vi "界面UI.vi"() -> ()   [LabVIEW 2016, in "超标留样集成.lvlib" / "德润DR803M超标留样.lvlib"]
uses:
  <vilib>/Utility/miscctls.llb/LVPointTypeDef.ctl
  <vilib>/Utility/config.llb/NI_LVConfig.lvlib
panel:
  out "String":string
  in  "超标测试":bool
  out "超标留样信号":bool
  out "留样结果":bool
  in  "协议选择":enum16{"原始协议", "MODBUS协议"}(ring)
  in  "设置":bool
  in  "工作进程":u16(ring) items=["停止中"=0, "启动延时"=1, "外置泵延时"=2, "管路润洗"=3, "管存"=4, "留样"=5, "出水管路排空"=6, "采水管路排空"=7, "待机"=13]
  out "采样器进程":i32(listbox)
  out "采样瓶数":u16
  out "留样模式":T1(ring)
  out "门状态":enum16{"门关", "门开"}(ring)
  out "仪器时间":timestamp format="%<%Y/%m/%d %H:%M:%S>T"
  out "当前瓶号":u16
  out "采样器状态":enum16{"停止", "运行", "系统初始化"}(ring)
  out "留样瓶满报警":bool
  out "超标留样等待时间/s":dbl
  in  "流程停止":bool
  in  "流程启动":bool
  out "流程中":bool
  out "VISA resource name":refnum<visa-resource-name>="COM10" caption="VISA资源名称"
  in  "采样启动":bool
  in  "切换运行":bool
  in  "时间校准":bool
  out "source":string
  out "通讯":bool
  # "只在待机时启动有效"
  # "德润超标留样803M"
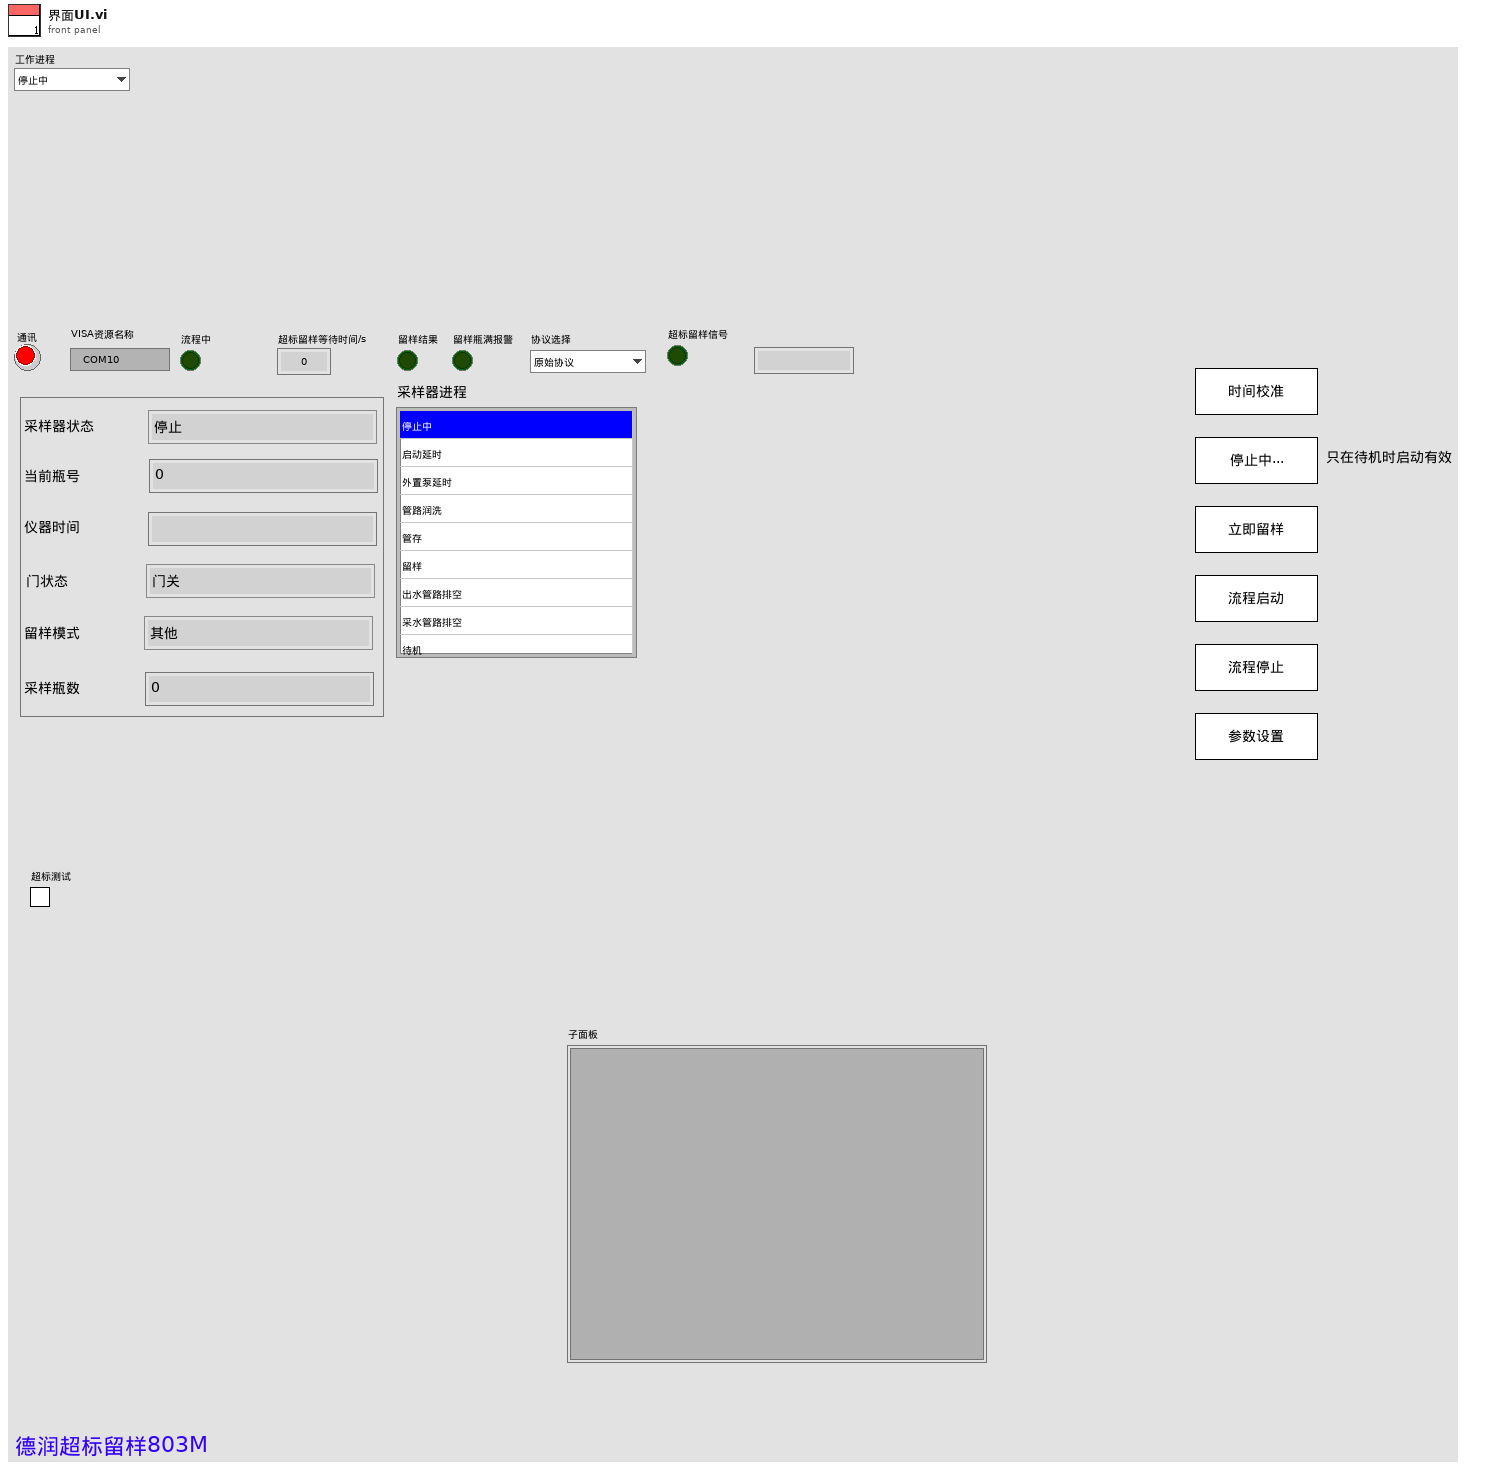
[diagram p1: front panel]
types:
  T1 = enum16{"其他", "定时留样", "时间等比例", "同步留样", "外控留样", "超标留样"}
  T2 = typedef "超标留样集成.lvlib/德润DR803M超标留样.lvlib/typedef.ctl" = cluster{"枚举":enum16{"open", "read", "write", "close", "write_register"}, "写入内容":string, "data_in":cluster{"write_coil_in":cluster{"address":u16, "value":bool}, "write_register_in":cluster{"address":u16, "values":u16[]}, "read_register_in":cluster{"starting address":u16, "quantity":u16}}}
  T3 = typedef "LVPointTypeDef.ctl" = cluster{"Horizontal":i16, "Vertical":i16}
  T4 = enum16{"打开串口", "写入", "读取", "关闭串口", "写入寄存器", "读取线圈"}
  T5 = cluster{"write_coil_in":cluster{"address":u16, "value":bool}, "write_register_in":cluster{"address":u16, "values":u16[]}, "read_register_in":cluster{"starting address":i32, "quantity":u16}}
  T6 = cluster{"write_coil_in":cluster{"address":u16, "value":bool}, "write_register_in":cluster{"address":u16, "values":u16[]}, "read_register_in":cluster{"starting address":u16, "quantity":u16}}[]
  T7 = cluster{"采样器状态":enum16{"停止", "运行", "系统初始化-2", "系统初始化-3", "初始化失败"}, "仪器时间":timestamp, "留样结果":bool, "工作模式":u16, "当前瓶号":u16, "平行样数":u16, "采样瓶数":u16, "设定每瓶采样次数":u16, "每瓶采样量":u16, "当前进程":u16, "当前瓶已采次数":u16, "留样中":bool}
  T8 = cluster{"仪器时间":timestamp, "工作状态":u16, "工作进程":u16, "采样模式":u16, "采样瓶数":dbl, "当前瓶号":dbl, "设定平行样数":dbl, "已采平行样":dbl, "设定每瓶采样次数":dbl, "已采次数":dbl, "当前瓶采样量":dbl, "瞬时流量":dbl, "累积流量":dbl, "混匀桶已采次数":dbl, "COD":dbl, "NH3N":dbl, "门状态":u16, "采样泵使能":dbl, "采样泵方向":dbl, "导流电机使能":dbl, "导流电机方向":dbl, "阀A":dbl, "阀B":dbl, "阀C":dbl, "外置泵":dbl, "预留":dbl}
  T9 = enum16{"停止", "运行", "系统初始化-2", "系统初始化-3", "初始化失败"}
  T10 = enum16{"open", "read", "write", "close", "write_register"}
  T11 = cluster{"write_coil_in":cluster{"address":u16, "value":bool}, "write_register_in":cluster{"address":u16, "values":u16[]}, "read_register_in":cluster{"starting address":u16, "quantity":u16}}
  T12 = typedef "LVDateTimeRec.ctl" = cluster{"秒数的小数部分":dbl, "秒":i32, "分":i32, "时":i32, "日":i32, "月":i32, "年":i32, "天数（周）":i32, "天数（年）":i32, "DST":i32}
  T13 = typedef "NI_LVConfig.lvlib/Config Data RefNum.ctl" = refnum<k1>
  T14 = enum32{"Bad", "Idle", "Run top level", "Running"}
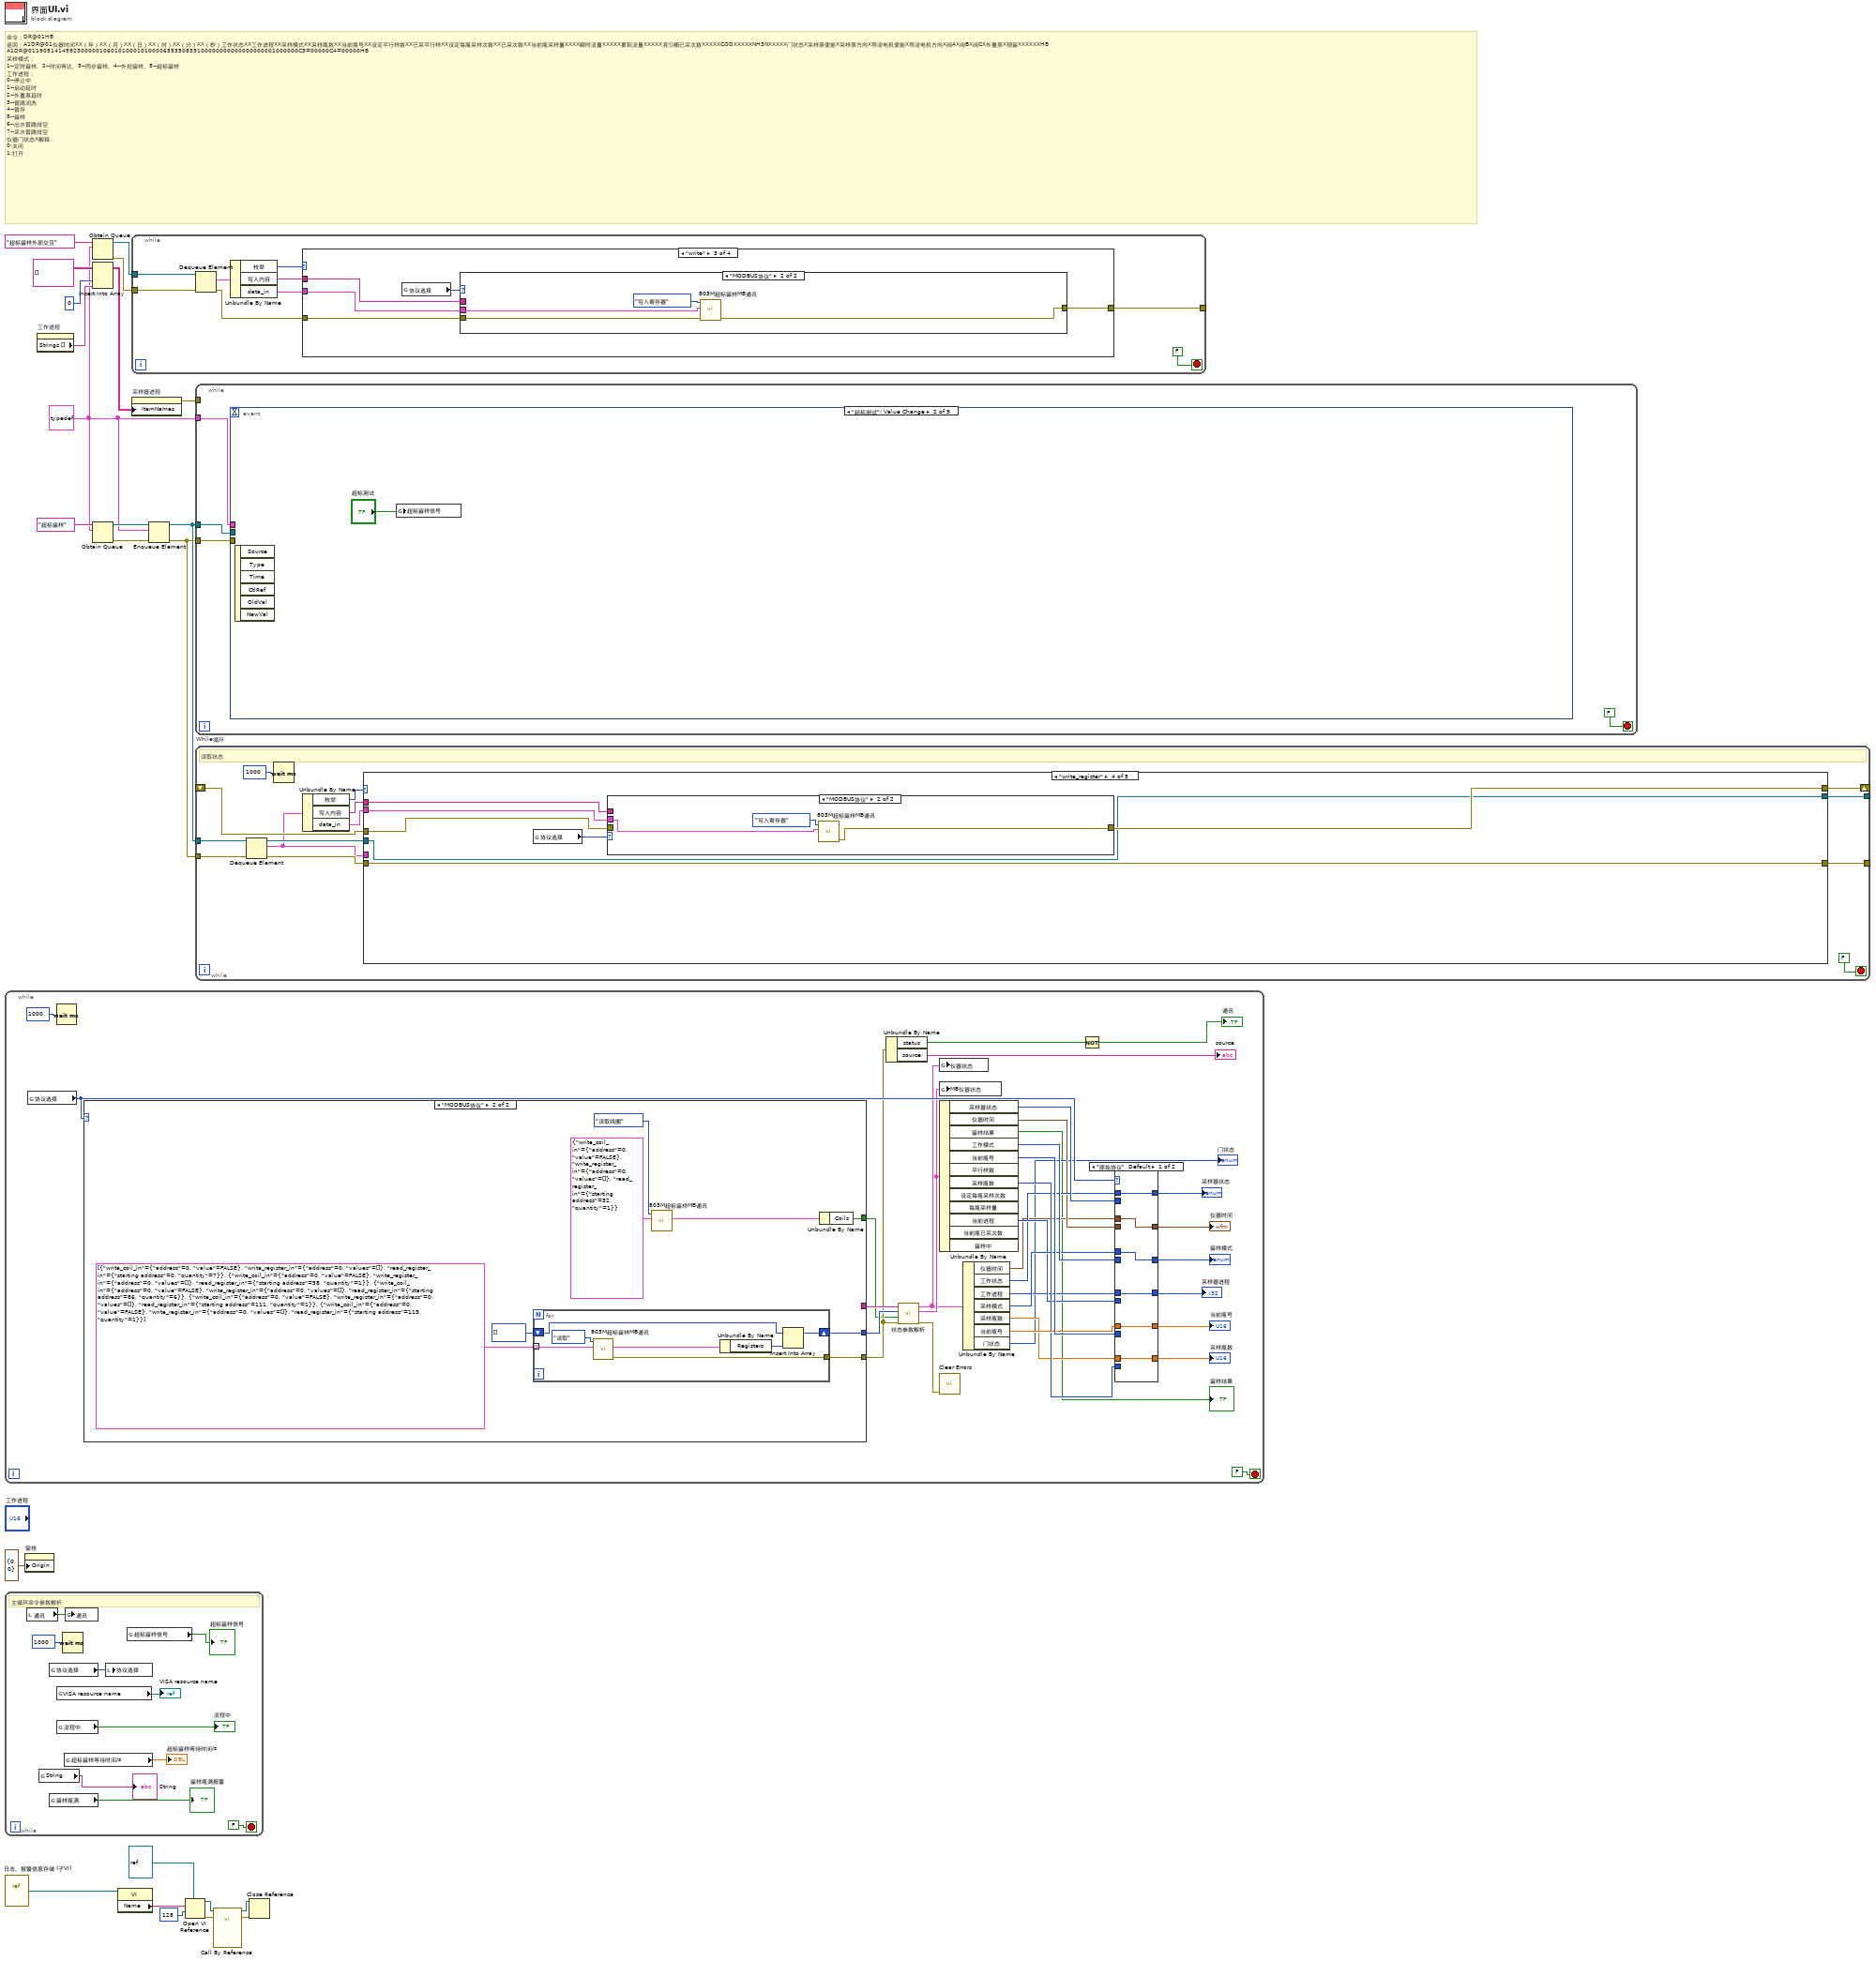
[diagram p0: block diagram]
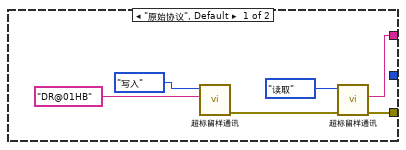
[diagram p3: hidden frame]
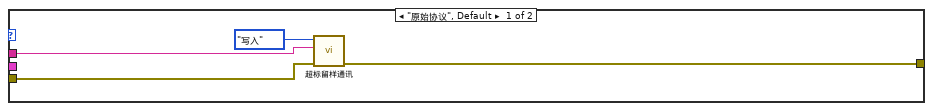
[diagram p6: hidden frame]
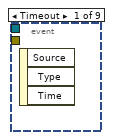
[diagram p8: hidden frame]
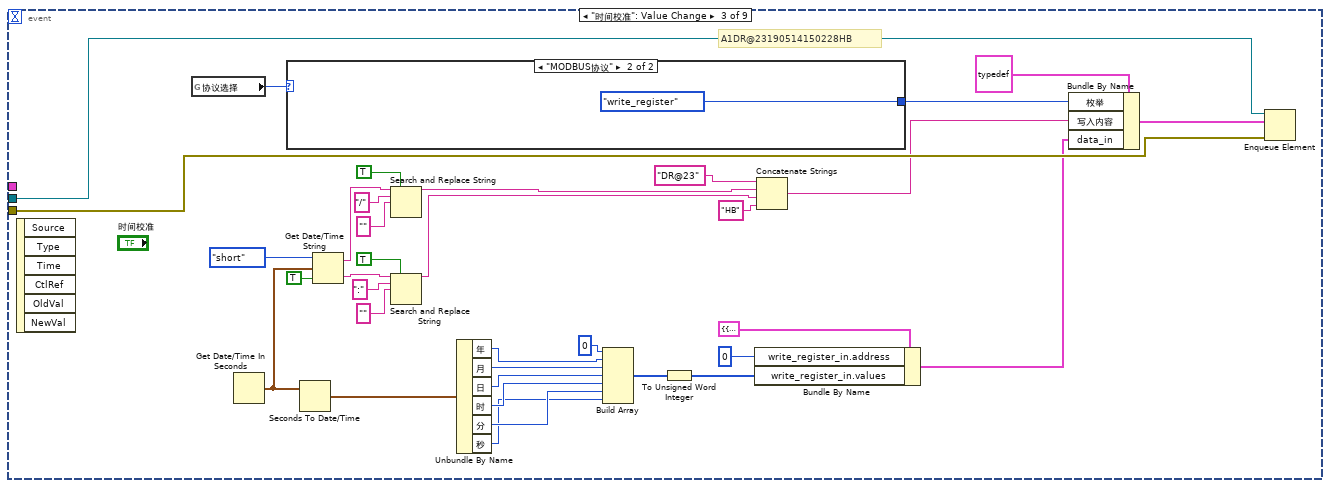
[diagram p9: hidden frame]
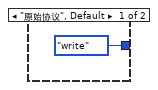
[diagram p10: hidden frame]
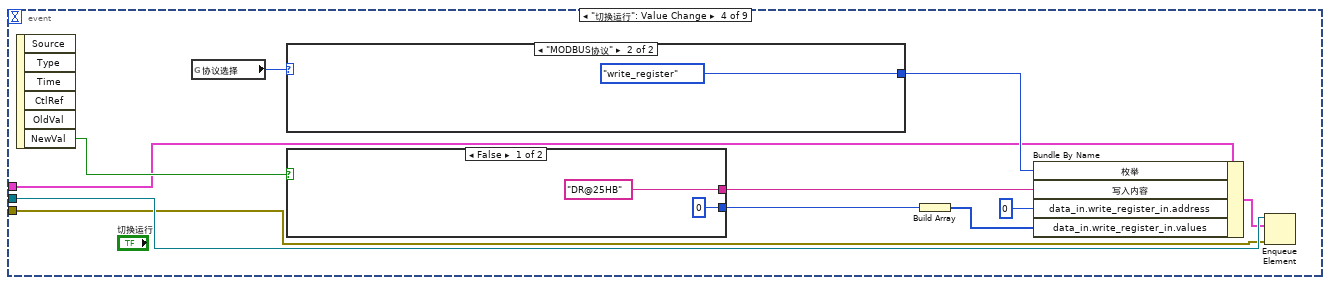
[diagram p11: hidden frame]
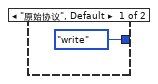
[diagram p12: hidden frame]
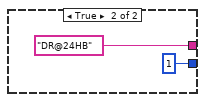
[diagram p13: hidden frame]
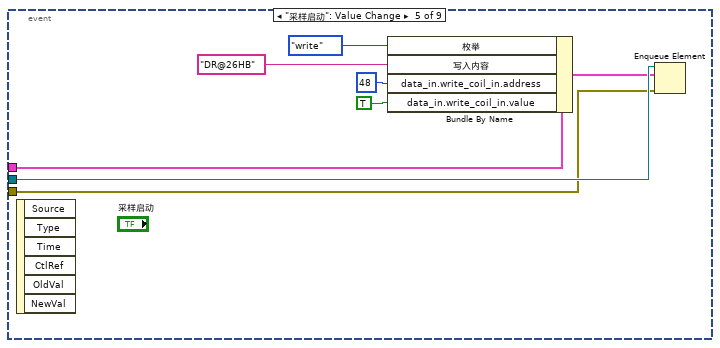
[diagram p14: hidden frame]
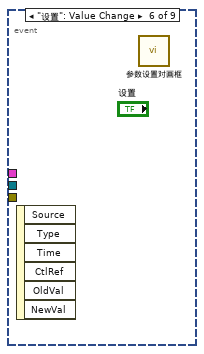
[diagram p15: hidden frame]
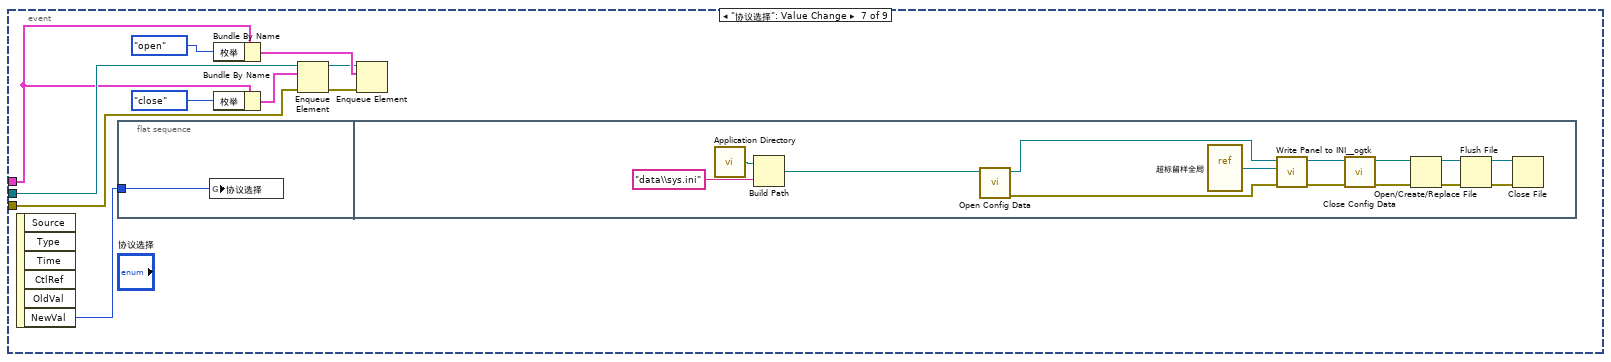
[diagram p16: hidden frame]
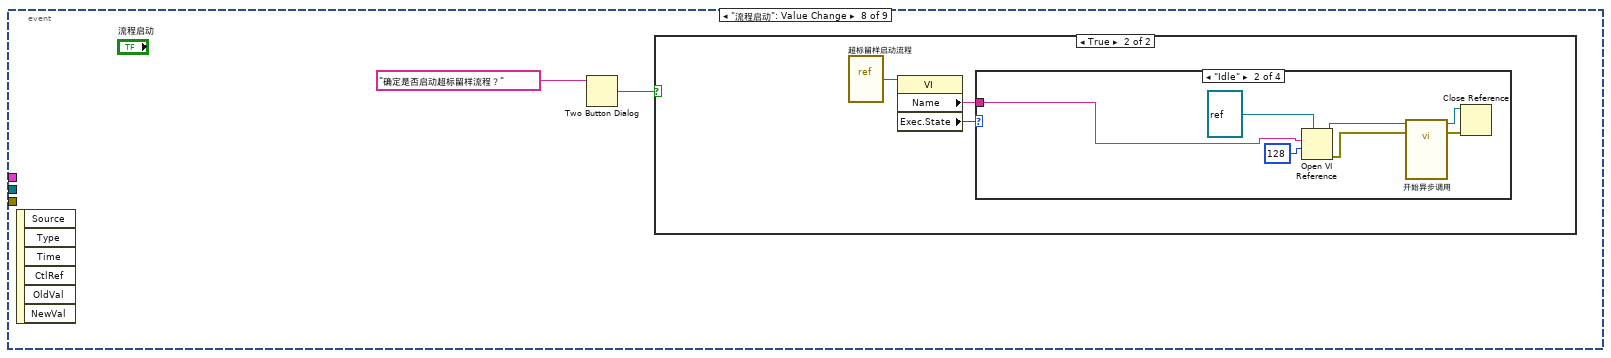
[diagram p17: hidden frame]
diagram:
  w1 = T2 {"枚举"=enum."open", "写入内容"="超标留样", "data_in"={"write_coil_in"={"address"=0, "value"=FALSE}, "write_register_in"={"address"=0, "values"=[]}, "read_register_in"={"starting address"=0, "quantity"=0}}}
  # "命令：DR@01HB\n返回：A1DR@01仪器时间XX（年）XX（月）XX（日）XX（时）XX（分）XX（秒）工作状态XX工作进程XX采样模式XX采样瓶数XX当前瓶号XX设定平行样数XX已采平行样XX设定每瓶采样次数XX已采次数XX当前瓶采样量XXXX瞬时流量XXXXX累积流量XXXXX混匀桶已采次数XXXXXCODXXXXXNH3NXXXXX门状态X采样泵使能X采样泵方向X导流电机使能X导流电机方向X阀AX阀BX阀CX外置泵X预留XXXXXXHB\nA1DR@011905141459230000010601010001010000655350839100000000000000000001000000C3=00000C4=00000HB\n采样模式：\n1--定时留样、2--时间等比、3--同步留样、4--外控留样、5--超标留样\n工作进程：\n0--停止中\n1--启动延时\n2--外置泵延时\n3--管路润洗\n4--管存\n5--留样\n6--出水管路排空\n7--采水管路排空\n仪器门状态X解释：\n0:关闭\n1:打开"
  n1 = while {
    stop <- FALSE stop-if-true
    n2 = global read "超标留样全局.vi" "协议选择"() -> (w39:enum16{"原始协议", "MODBUS协议"})
    n3 = Wait (ms)(milliseconds to wait=u32 1000 ("等待时间（毫秒）")) -> ()  [unwired: 1 out]
    n4 = case shown="\"MODBUS协议\"" w39 {
      tunnel: [w73 w79] -> w27
      tunnel: [w72 _] -> w28
      tunnel: [_ w80] -> w34
      tunnel: [_ w75] -> w24
      frame "原始协议", Default {
        n5 = call "超标留样通讯.vi"("写入缓冲区"="DR@01HB", "功能输入"=enum16{"打开串口", "写入", "读取", "关闭串口"}."写入") -> ("error out"=w74:errorcluster)  [unwired: 7 in, 2 out]
        n6 = call "超标留样通讯.vi"("error in (no error)"=w74, "功能输入"=enum16{"打开串口", "写入", "读取", "关闭串口"}."读取") -> ("error out"=w73:errorcluster, "读取缓冲区"=w72:string)  [unwired: 7 in, 1 out]
      }
      frame "MODBUS协议" {
        n7 = for {
          shift-right: [w86] -> w80
          shift-left: u16[] [] -> [w85]
          tunnel: T6 [{"write_coil_in"={"address"=0, "value"=FALSE}, "write_register_in"={"address"=0, "values"=[]}, "read_register_in"={"starting address"=0, "quantity"=7}}, {"write_coil_in"={"address"=0, "value"=FALSE}, "write_register_in"={"address"=0, "values"=[]}, "read_register_in"={"starting address"=58, "quantity"=1}}, {"write_coil_in"={"address"=0, "value"=FALSE}, "write_register_in"={"address"=0, "values"=[]}, "read_register_in"={"starting address"=86, "quantity"=6}}, {"write_coil_in"={"address"=0, "value"=FALSE}, "write_register_in"={"address"=0, "values"=[]}, "read_register_in"={"starting address"=111, "quantity"=1}}, {"write_coil_in"={"address"=0, "value"=FALSE}, "write_register_in"={"address"=0, "values"=[]}, "read_register_in"={"starting address"=115, "quantity"=1}}] -> [w84] mode=indexing
          tunnel: [w83] -> w79
          n8 = call "803M超标留样MB通讯.vi"("data_in"=w84, "功能输入"=T4."读取") -> ("error out"=w83:errorcluster, "data_out"=w88:cluster{"Registers":u16[], "Coils":bool[]})  [unwired: 8 in]
          n9 = Unbundle By Name(w88) -> ("Registers"=w87:u16[])
          n10 = Insert Into Array(array=w85, new element=w87) -> (w86:u16[])  [unwired: 1 in]
        }
        n11 = call "803M超标留样MB通讯.vi"("data_in"=T5 {"write_coil_in"={"address"=0, "value"=FALSE}, "write_register_in"={"address"=0, "values"=[]}, "read_register_in"={"starting address"=32, "quantity"=1}}, "功能输入"=T4."读取线圈") -> ("data_out"=w76:cluster{"Registers":u16[], "Coils":bool[]})  [unwired: 8 in, 1 out]
        n12 = Unbundle By Name(w76) -> ("Coils"=w75:bool[])
      }
    }
    n13 = Unbundle By Name(w27) -> ("status"=w29:bool, "source"=→"source":string)
    n14 = call "状态参数解析.vi"("error in (no error)"=w27, "Coils"=w24, "数组"=w34, "字符串"=w28) -> ("error out"=w33:errorcluster, "簇 2"=w35:T7, "簇"=w32:T8)  [unwired: 5 in]
    n15 = global write "超标留样全局.vi" "仪器状态"(w32) -> ()
    n16 = global write "超标留样全局.vi" "MB仪器状态"(w35) -> ()
    n17 = Unbundle By Name(w35) -> ("采样器状态"=w43:T9, "仪器时间"=w40:timestamp, "留样结果"=→"留样结果":bool, "工作模式"=w49:u16, "当前瓶号"=w55:u16, "采样瓶数"=w52:u16, "当前进程"=w46:u16)  [unwired: 5 out]
    n18 = call <vilib>:"Clear Errors.vi"("error in (no error)"=w33) -> ()  [unwired: 5 in, 2 out]
    n19 = Unbundle By Name(w32) -> ("仪器时间"=w37:timestamp, "工作状态"=w41:u16, "工作进程"=w44:u16, "采样模式"=w47:u16, "采样瓶数"=w50:dbl, "当前瓶号"=w53:dbl, "门状态"=→"门状态":u16)
    n20 = Not(x=w29) -> (.not. x?=→"通讯":bool)
    n21 = case shown="\"原始协议\", Default" w39 {
      tunnel: w37 -> [w62 _]
      tunnel: [w62 w68] -> w38
      tunnel: w40 -> [_ w68]
      tunnel: w41 -> [w61 _]
      tunnel: [w61 w67] -> w42
      tunnel: w43 -> [_ w67]
      tunnel: w44 -> [w60 _]
      tunnel: [w60 w66] -> w45
      tunnel: w46 -> [_ w66]
      tunnel: w47 -> [w59 _]
      tunnel: [w59 w65] -> w48
      tunnel: w49 -> [_ w65]
      tunnel: w50 -> [w58 _]
      tunnel: [w58 w64] -> w51
      tunnel: w52 -> [_ w64]
      tunnel: w53 -> [w57 _]
      tunnel: [w57 w63] -> w54
      tunnel: w55 -> [_ w63]
      frame "原始协议", Default {
      }
      frame "MODBUS协议" {
      }
    }
    "仪器时间" <- w38
    "采样器状态" <- w42
    "当前瓶号" <- w54
    "留样模式" <- w48
    "采样瓶数" <- w51
    "采样器进程" <- w45
  }
  n22 = while {
    stop <- FALSE stop-if-true
    # "主循环命令参数解析"
    n23 = local read "通讯"() -> (w97:bool)
    n24 = global read "超标留样全局.vi" "String"() -> (→"String":string)
    n25 = global read "超标留样全局.vi" "协议选择"() -> (w92:enum16{"原始协议", "MODBUS协议"})
    n26 = global read "超标留样全局.vi" "留样瓶满"() -> (→"留样瓶满报警":bool)
    n27 = global read "超标留样全局.vi" "VISA resource name"() -> (→"VISA resource name":refnum<visa-resource-name>)
    n28 = global read "超标留样全局.vi" "流程中"() -> (→"流程中":bool)
    n29 = Wait (ms)(milliseconds to wait=u32 1000 ("等待时间（毫秒）")) -> ()  [unwired: 1 out]
    n30 = global read "超标留样全局.vi" "超标留样等待时间/s"() -> (→"超标留样等待时间/s":dbl)
    n31 = global write "超标留样全局.vi" "通讯"(w97) -> ()
    n32 = local write "协议选择"(w92) -> ()
    n33 = global read "超标留样全局.vi" "超标留样信号"() -> (→"超标留样信号":bool)
  }
  n34 = vi-ref "日志、报警信息存储 (子VI).vi"() -> (w14:refnum<vi>)
  n35 = property on="窗格" class="Pane"("Origin"=T3 {"Horizontal"=0, "Vertical"=0} ("原点")) -> ()  [unwired: 2 in, 2 out]
  n36 = property on="工作进程" class="Ring (strict)"() -> ("Strings []"=w4:string[])  [unwired: 2 in, 2 out]
  n37 = Obtain Queue(name (unnamed)="超标留样外部交互" ("名称（未命名）"), element data type=w1) -> (queue out=w16:refnum<queue>, error out=w15:errorcluster)  [unwired: 3 in, 1 out]
  n38 = Insert Into Array(array=string[][] [] ("字符串[]"), index (col)=0 ("禁用的索引 (列)"), new element=w4) -> (w3:string[][])  [unwired: 1 in]
  n39 = Obtain Queue(name (unnamed)="超标留样" ("名称（未命名）"), element data type=w1) -> (queue out=w22:refnum<queue>, error out=w21:errorcluster)  [unwired: 3 in, 1 out]
  n40 = property class="VI"(reference=w14) -> ("Name"=w13:string)  [unwired: 1 in, 2 out]
  n41 = while {
    tunnel: w16 -> [w108]
    tunnel: w15 -> [w107]
    tunnel: [w101] -> _
    stop <- FALSE stop-if-true
    n42 = Dequeue Element(queue=w108, error in (no error)=w107) -> (element=w105:T2, error out=w102:errorcluster)  [unwired: 1 in, 2 out]
    n43 = Unbundle By Name(w105) -> ("枚举"=w104:T10, "写入内容"=w103:string, "data_in"=w100:T11)
    n44 = case shown="\"write\"" w104 {
      tunnel: w103 -> [_ _ w113 _]
      tunnel: w102 -> [_ _ w112 _]
      tunnel: [_ _ w111 _] -> w101
      tunnel: w100 -> [_ _ w109 _]
      frame "open", Default {
      }
      frame "read" {
      }
      frame "write" {
        n45 = global read "超标留样全局.vi" "协议选择"() -> (w110:enum16{"原始协议", "MODBUS协议"})
        n46 = case shown="\"MODBUS协议\"" w110 {
          tunnel: w113 -> [w117 _]
          tunnel: w112 -> [w115 w119]
          tunnel: [w114 w118] -> w111
          tunnel: w109 -> [_ w120]
          frame "原始协议", Default {
            n47 = call "超标留样通讯.vi"("error in (no error)"=w115, "写入缓冲区"=w117, "功能输入"=enum16{"打开串口", "写入", "读取", "关闭串口"}."写入") -> ("error out"=w114:errorcluster)  [unwired: 6 in, 2 out]
          }
          frame "MODBUS协议" {
            n48 = call "803M超标留样MB通讯.vi"("error in (no error)"=w119, "data_in"=w120, "功能输入"=enum16{"打开串口", "写入", "读取", "关闭串口", "写入寄存器"}."写入寄存器") -> ("error out"=w118:errorcluster)  [unwired: 7 in, 1 out]
          }
        }
      }
      frame "close" {
      }
    }
  }
  n49 = property on="采样器进程" class="MCListbox (strict)"("ItemNames"=w3) -> (error out=w2:errorcluster)  [unwired: 2 in, 1 out]
  n50 = Enqueue Element(queue=w22, element=w1, error in (no error)=w21) -> (queue out=w20:refnum<queue>, error out=w19:errorcluster)  [unwired: 1 in, 1 out]
  n51 = Open VI Reference(type specifier VI Refnum (for type only)=refnum<vi> refnum ("类型说明符VI引用句柄（仅用于类型）"), vi path=w13, options=128 ("选项")) -> (vi reference=w11:refnum<vi>, error out=w9:errorcluster)  [unwired: 3 in]
  n52 = while {
    tunnel: w20 -> [w124]
    tunnel: w19 -> [w123]
    tunnel: w2 -> [_]
    tunnel: w1 -> [w122]
    stop <- FALSE stop-if-true
    n53 = event shown="[1] \"超标测试\": Value Change" {
      selector: _ -> [_ _ _ _ _ _ _ _ _]
      dyn-events: _ -> [_ _ _ _ _ _ _ _ _]
      timeout: _ -> [_ _ _ _ _ _ _ _ _]
      tunnel: w124 -> [_ _ w161 w174 w188 _ w194 _ w228]
      tunnel: w123 -> [_ _ w160 w173 w187 _ w192 _ w227]
      tunnel: w122 -> [_ _ _ w168 w184 _ w193 _ w226]
      event Timeout {
        n54 = event-data() -> ()  [unwired: 1 in, 3 out]
      }
      event "超标测试": Value Change {
        n55 = event-data() -> ()  [unwired: 1 in, 6 out]
        n56 = global write "超标留样全局.vi" "超标留样信号"("超标测试") -> ()
      }
      event "时间校准": Value Change {
        # "A1DR@23190514150228HB"
        n57 = event-data() -> ()  [unwired: 1 in, 6 out]
        n58 = global read "超标留样全局.vi" "协议选择"() -> (w141:enum16{"原始协议", "MODBUS协议"})
        n59 = Get Date/Time In Seconds() -> (seconds since 1Jan1904=w138:timestamp)
        n60 = case shown="\"MODBUS协议\"" w141 {
          tunnel: [T10."write" ("枚举") T10."write_register" ("枚举")] -> w140
          frame "原始协议", Default {
          }
          frame "MODBUS协议" {
          }
        }
        n61 = Seconds To Date/Time(time stamp (now)=w138) -> (date time rec=w137:T12)  [unwired: 1 in]
        n62 = Get Date/Time String(date format (0)=enum16{"short", "long", "abbreviated"}."short" ("日期格式(0)"), seconds (now)=w138, want seconds? (F)=TRUE ("需要秒？(F)")) -> (date string=w156:string, time string=w149:string)
        n63 = Search and Replace String(replace all?=TRUE ("替换全部？(F)"), input string=w156, search string="/" ("搜索字符串"), replace string="" ("替换字符串(\"\")")) -> (result string=w148:string)  [unwired: 4 in, 3 out]
        n64 = Search and Replace String(replace all?=TRUE ("替换全部？(F)"), input string=w149, search string=":" ("搜索字符串"), replace string="" ("替换字符串(\"\")")) -> (result string=w147:string)  [unwired: 4 in, 3 out]
        n65 = Unbundle By Name(w137) -> ("年"=w136:i32, "月"=w135:i32, "日"=w134:i32, "时"=w133:i32, "分"=w132:i32, "秒"=w131:i32)
        n66 = Build Array(0 ("元素"), w136, w135, w134, w133, w132, w131) -> (w130:i32[])
        n67 = To Unsigned Word Integer(number=w130) -> (unsigned 16bit integer=w128:u16[])
        n68 = Bundle By Name(cluster=T11 {"write_coil_in"={"address"=0, "value"=FALSE}, "write_register_in"={"address"=0, "values"=[]}, "read_register_in"={"starting address"=0, "quantity"=0}} ("data_in"), "write_register_in.address"=u16 0, "write_register_in.values"=w128) -> (w139:T11)
        n69 = Concatenate Strings("DR@23" ("写入缓冲区"), w148, w147, "HB" ("写入缓冲区")) -> (w144:string)
        n70 = Bundle By Name(cluster=T2 {"枚举"=enum."open", "写入内容"="超标留样", "data_in"={"write_coil_in"={"address"=0, "value"=FALSE}, "write_register_in"={"address"=0, "values"=[]}, "read_register_in"={"starting address"=0, "quantity"=0}}}, "枚举"=w140, "写入内容"=w144, "data_in"=w139) -> (w145:T2)
        n71 = Enqueue Element(queue=w161, element=w145, error in (no error)=w160) -> ()  [unwired: 1 in, 3 out]
      }
      event "切换运行": Value Change {
        n72 = event-data() -> ("NewVal"=w172:bool)  [unwired: 1 in, 5 out]
        n73 = global read "超标留样全局.vi" "协议选择"() -> (w167:enum16{"原始协议", "MODBUS协议"})
        n74 = case shown="\"MODBUS协议\"" w167 {
          tunnel: [T10."write" ("枚举") T10."write_register" ("枚举")] -> w171
          frame "原始协议", Default {
          }
          frame "MODBUS协议" {
          }
        }
        n75 = case shown="False" w172 {
          tunnel: ["DR@25HB" ("写入缓冲区") "DR@24HB"] -> w170
          tunnel: [u16 0 ("value") u16 1 ("value")] -> w165
          frame False {
          }
          frame True {
          }
        }
        n76 = Build Array(w165) -> (w164:u16[])
        n77 = Bundle By Name(cluster=w168, "枚举"=w171, "写入内容"=w170, "data_in.write_register_in.address"=u16 0, "data_in.write_register_in.values"=w164) -> (w169:T2)
        n78 = Enqueue Element(queue=w174, element=w169, error in (no error)=w173) -> ()  [unwired: 1 in, 3 out]
      }
      event "采样启动": Value Change {
        n79 = event-data() -> ()  [unwired: 1 in, 6 out]
        n80 = Bundle By Name(cluster=w184, "枚举"=enum16{"open", "read", "write", "close"}."write" ("元素"), "写入内容"="DR@26HB", "data_in.write_coil_in.address"=u16 48, "data_in.write_coil_in.value"=TRUE) -> (w185:T2)
        n81 = Enqueue Element(queue=w188, element=w185, error in (no error)=w187) -> ()  [unwired: 1 in, 3 out]
      }
      event "设置": Value Change {
        n82 = event-data() -> ()  [unwired: 1 in, 6 out]
        n83 = call "参数设置对画框.vi"() -> ()  [unwired: 12 in]
      }
      event "协议选择": Value Change {
        n84 = event-data() -> ("NewVal"=w189:enum16{"原始协议", "MODBUS协议"})  [unwired: 1 in, 5 out]
        n85 = flat-sequence {
          tunnel: w189 -> [w199]
          frame #0 {
            n86 = global write "超标留样全局.vi" "协议选择"(w199) -> ()
          }
          frame #1 {
            n87 = call <vilib>:"Application Directory.vi"() -> ("Application Directory"=w201:path)
            n88 = Build Path(base path=w201, name or relative path="data\\sys.ini" ("名称或相对路径")) -> (appended path=w202:path)
            n89 = call <vilib>:"Open Config Data.vi"("configuration file path"=w202) -> ("error out"=w206:errorcluster, "refnum"=w203:T13)  [unwired: 8 in, 1 out]
            n90 = vi-ref "超标留样全局.vi"() -> (w204:refnum<vi>)
            n91 = call <userlib>:"Write Panel to INI__ogtk.vi"("error in (no error)"=w206, "VI ref"=w204, "refnum"=w203) -> ("error out"=w207:errorcluster, "refnum out"=w205:T13)  [unwired: 7 in]
            n92 = call <vilib>:"Close Config Data.vi"("error in (no error)"=w207, "refnum"=w205) -> ("error out"=w212:errorcluster, "file path"=w213:path)  [unwired: 8 in]
            n93 = Open/Create/Replace File(file path (use dialog)=w213, error in=w212) -> (refnum out=w209:refnum<file>, error out=w208:errorcluster)  [unwired: 4 in, 1 out]
            n94 = Flush File(refnum=w209, error in=w208) -> (refnum out=w210:refnum<file>, error out=w211:errorcluster)
            n95 = Close File(refnum=w210, error in=w211) -> ()  [unwired: 2 out]
          }
        }
        n96 = Bundle By Name(cluster=w193, "枚举"=T10."open") -> (w197:T2)
        n97 = Bundle By Name(cluster=w193, "枚举"=T10."close") -> (w198:T2)
        n98 = Enqueue Element(queue=w194, element=w198, error in (no error)=w192) -> (queue out=w196:refnum<queue>, error out=w195:errorcluster)  [unwired: 1 in, 1 out]
        n99 = Enqueue Element(queue=w196, element=w197, error in (no error)=w195) -> ()  [unwired: 1 in, 3 out]
      }
      event "流程启动": Value Change {
        n100 = event-data() -> ()  [unwired: 1 in, 6 out]
        n101 = Two Button Dialog(message="确定是否启动超标留样流程？" ("消息")) -> (T button?=w214:bool)  [unwired: 2 in]
        n102 = case shown="True" w214 {
          frame False {
          }
          frame True {
            n103 = vi-ref "超标留样启动流程.vi"() -> (w216:refnum<vi>)
            n104 = property class="VI"(reference=w216) -> ("Name"=w217:string, "Exec.State"=w218:T14)  [unwired: 1 in, 2 out]
            n105 = case shown="\"Idle\"" w218 {
              tunnel: w217 -> [_ w221 _ _]
              frame "Bad", Default {
              }
              frame "Idle" {
                n106 = Open VI Reference(type specifier VI Refnum (for type only)=refnum<vi> refnum ("类型说明符VI引用句柄（仅用于类型）"), vi path=w221, options=128 ("选项")) -> (vi reference=w225:refnum<vi>, error out=w220:errorcluster)  [unwired: 3 in]
                n107 = call-by-ref "开始异步调用"(reference=w225, error in=w220) -> (reference out=w224:refnum<vi>, error out=w219:errorcluster)  [unwired: 12 in]
                n108 = Close Reference(reference=w224, error in (no error)=w219) -> ()  [unwired: 1 out]
              }
              frame "Run top level" {
              }
              frame "Running" {
              }
            }
          }
        }
      }
      event "流程停止": Value Change {
        n109 = event-data() -> ()  [unwired: 1 in, 6 out]
        n110 = Two Button Dialog(message="确定是否停止超标留样流程并排空当前瓶？" ("消息")) -> (T button?=w229:bool)  [unwired: 2 in]
        n111 = case shown="True" w229 {
          tunnel: w228 -> [_ w239]
          tunnel: w227 -> [_ w238]
          tunnel: w226 -> [_ w235]
          frame False {
          }
          frame True {
            n112 = global read "超标留样全局.vi" "协议选择"() -> (w234:enum16{"原始协议", "MODBUS协议"})
            n113 = case shown="\"原始协议\", Default" w234 {
              tunnel: [T10."write" ("枚举") T10."write_register" ("枚举")] -> w233
              frame "原始协议", Default {
              }
              frame "MODBUS协议" {
              }
            }
            n114 = Obtain Notifier(name (unnamed)="超标留样流程" ("名称（未命名）"), notification data type=FALSE ("采样完成")) -> (notifier out=w244:refnum<notifier>, error out=w243:errorcluster)  [unwired: 2 in, 1 out]
            n115 = Send Notification(notification=TRUE ("通知"), notifier=w244, error in (no error)=w243) -> (notifier out=w241:refnum<notifier>, error out=w240:errorcluster)
            n116 = Release Notifier(notifier=w241, error in (no error)=w240) -> ()  [unwired: 1 in, 3 out]
            n117 = Bundle By Name(cluster=w235, "枚举"=w233, "写入内容"="DR@25HB" ("写入缓冲区"), "data_in.write_register_in.address"=u16 0, "data_in.write_register_in.values"=u16[] [0]) -> (w236:T2)
            n118 = Enqueue Element(queue=w239, element=w236, error in (no error)=w238) -> ()  [unwired: 1 in, 3 out]
          }
        }
      }
    }
  }
  n119 = while "While循环" {
    tunnel: w20 -> [w260]
    tunnel: w19 -> [w259]
    tunnel: [w256] -> _
    tunnel: [w255] -> _
    shift-right: [w253] -> _
    shift-left: _ -> [w254]
    stop <- FALSE stop-if-true
    # "读取状态"
    n120 = Dequeue Element(queue=w260, error in (no error)=w259) -> (queue out=w258:refnum<queue>, element=w249:T2, error out=w257:errorcluster)  [unwired: 1 in, 1 out]
    n121 = Wait (ms)(milliseconds to wait=u32 1000 ("等待时间（毫秒）")) -> ()  [unwired: 1 out]
    n122 = Unbundle By Name(w249) -> ("枚举"=w252:T10, "写入内容"=w251:string, "data_in"=w250:T11)
    n123 = case shown="\"write_register\"" w252 {
      tunnel: [w267 w279 w315 w329 w341] -> w253
      tunnel: w258 -> [w266 w278 w311 w325 w340]
      tunnel: w257 -> [w265 w277 w310 w324 w339]
      tunnel: [w266 w278 w311 w325 w340] -> w256
      tunnel: [w265 w277 w310 w324 w339] -> w255
      tunnel: w254 -> [_ w280 w316 w330 w342]
      tunnel: w251 -> [_ w276 w314 w328 _]
      tunnel: w250 -> [_ w274 w312 w326 _]
      tunnel: w249 -> [_ _ _ _ _]
      frame "open", Default {
        n124 = global read "超标留样全局.vi" "VISA resource name"() -> (w264:refnum<visa-resource-name>)
        n125 = global read "超标留样全局.vi" "协议选择"() -> (w263:enum16{"原始协议", "MODBUS协议"})
        n126 = case shown="\"MODBUS协议\"" w263 {
          tunnel: [w269 w271] -> w267
          tunnel: w264 -> [w268 w272]
          frame "原始协议", Default {
            n127 = call "超标留样通讯.vi"("VISA resource name"=w268, "功能输入"=enum16{"打开串口", "写入", "读取", "关闭串口"}."打开串口") -> ("error out"=w269:errorcluster)  [unwired: 7 in, 2 out]
          }
          frame "MODBUS协议" {
            n128 = call "803M超标留样MB通讯.vi"("VISA resource name"=w272, "功能输入"=enum16{"打开串口", "写入", "读取", "关闭串口", "写入寄存器"}."打开串口") -> ("error out"=w271:errorcluster)  [unwired: 8 in, 1 out]
          }
        }
      }
      frame "read" {
        n129 = global read "超标留样全局.vi" "协议选择"() -> (w275:enum16{"原始协议", "MODBUS协议"})
        n130 = case shown="\"MODBUS协议\"" w275 {
          tunnel: w280 -> [w285 w307]
          tunnel: [w284 w306] -> w279
          tunnel: w276 -> [w282 _]
          tunnel: w274 -> [_ w308]
          frame "原始协议", Default {
            n131 = call "超标留样通讯.vi"("error in (no error)"=w285, "功能输入"=enum16{"打开串口", "写入", "读取", "关闭串口"}."读取") -> ("error out"=w284:errorcluster, "读取缓冲区"=w283:string)  [unwired: 7 in, 1 out]
            n132 = case shown="\"DR@58HB\"" w282 {
              tunnel: w283 -> [w286 w293 w300]
              frame "DR@16HB" {
                n133 = flat-sequence {
                  tunnel: w286 -> [w289]
                  frame #0 {
                    n134 = call "超标留样状态参数解析.vi"("输入字符串"=w289, "解析/转指令"=enum16{"解析", "转指令"}."解析", "模式选择"=enum16{"外控留样", "超标留样"}."超标留样") -> ()  [unwired: 11 in, 2 out]
                  }
                  frame #1 {
                    n135 = global write "超标留样全局.vi" "读取更新"(TRUE ("读取更新")) -> ()
                  }
                  frame #2 {
                    n136 = Wait (ms)(milliseconds to wait=u32 500 ("等待时间（毫秒）")) -> ()  [unwired: 1 out]
                  }
                  frame #3 {
                    n137 = global write "超标留样全局.vi" "读取更新"(FALSE ("读取更新")) -> ()
                  }
                }
              }
              frame "DR@58HB" {
                n138 = flat-sequence {
                  tunnel: w293 -> [w294]
                  frame #0 {
                    n139 = call "超标留样状态参数解析.vi"("输入字符串"=w294, "解析/转指令"=enum16{"解析", "转指令"}."解析", "模式选择"=enum16{"外控留样", "超标留样"}."外控留样") -> ()  [unwired: 11 in, 2 out]
                  }
                  frame #1 {
                    n140 = global write "超标留样全局.vi" "外控留样读取更新"(TRUE ("读取更新")) -> ()
                  }
                  frame #2 {
                    n141 = Wait (ms)(milliseconds to wait=u32 500 ("等待时间（毫秒）")) -> ()  [unwired: 1 out]
                  }
                  frame #3 {
                    n142 = global write "超标留样全局.vi" "外控留样读取更新"(FALSE ("读取更新")) -> ()
                  }
                }
              }
              frame "超标留样设置", Default {
                n143 = disable-structure shown="禁用" {
                  disable-tunnel: w300 -> [w305 _]
                  frame Disabled {
                    n144 = String Subset(string=w305, offset (0)=5 ("偏移量(0)")) -> (substring=w303:string)  [unwired: 1 in]
                    n145 = Search/Split String(string=w303, search string/char (-)="HB" ("搜索字符串/字符(-)")) -> (substring before match=w301:string)  [unwired: 1 in, 2 out]
                    n146 = One Button Dialog(message=w301) -> ()  [unwired: 1 in, 1 out]
                  }
                  frame Enabled {
                  }
                }
              }
            }
          }
          frame "MODBUS协议" {
            n147 = call "803M超标留样MB通讯.vi"("error in (no error)"=w307, "data_in"=w308, "功能输入"=enum16{"打开串口", "写入", "读取", "关闭串口", "写入寄存器"}."读取") -> ("error out"=w306:errorcluster)  [unwired: 7 in, 1 out]
          }
        }
      }
      frame "write" {
        n148 = global read "超标留样全局.vi" "协议选择"() -> (w313:enum16{"原始协议", "MODBUS协议"})
        n149 = case shown="\"MODBUS协议\"" w313 {
          tunnel: w316 -> [w320 _]
          tunnel: [w319 w322] -> w315
          tunnel: w314 -> [w317 _]
          tunnel: w312 -> [_ w321]
          frame "原始协议", Default {
            n150 = call "超标留样通讯.vi"("error in (no error)"=w320, "写入缓冲区"=w317, "功能输入"=enum16{"打开串口", "写入", "读取", "关闭串口"}."写入") -> ("error out"=w319:errorcluster)  [unwired: 6 in, 2 out]
          }
          frame "MODBUS协议" {
            n151 = call "803M超标留样MB通讯.vi"("data_in"=w321, "功能输入"=enum16{"打开串口", "写入", "读取", "关闭串口", "写入寄存器"}."写入") -> ("error out"=w322:errorcluster)  [unwired: 8 in, 1 out]
          }
        }
      }
      frame "write_register" {
        n152 = global read "超标留样全局.vi" "协议选择"() -> (w327:enum16{"原始协议", "MODBUS协议"})
        n153 = case shown="\"MODBUS协议\"" w327 {
          tunnel: w330 -> [w334 _]
          tunnel: [w333 w336] -> w329
          tunnel: w328 -> [w331 _]
          tunnel: w326 -> [_ w335]
          frame "原始协议", Default {
            n154 = call "超标留样通讯.vi"("error in (no error)"=w334, "写入缓冲区"=w331, "功能输入"=enum16{"打开串口", "写入", "读取", "关闭串口"}."写入") -> ("error out"=w333:errorcluster)  [unwired: 6 in, 2 out]
          }
          frame "MODBUS协议" {
            n155 = call "803M超标留样MB通讯.vi"("data_in"=w335, "功能输入"=enum16{"打开串口", "写入", "读取", "关闭串口", "写入寄存器"}."写入寄存器") -> ("error out"=w336:errorcluster)  [unwired: 8 in, 1 out]
          }
        }
      }
      frame "close" {
        n156 = global read "超标留样全局.vi" "协议选择"() -> (w338:enum16{"原始协议", "MODBUS协议"})
        n157 = case shown="\"MODBUS协议\"" w338 {
          tunnel: w342 -> [w345 w346]
          tunnel: [w343 w347] -> w341
          frame "原始协议", Default {
            n158 = call "超标留样通讯.vi"("error in (no error)"=w345, "功能输入"=enum16{"打开串口", "写入", "读取", "关闭串口"}."关闭串口") -> ("error out"=w343:errorcluster)  [unwired: 7 in, 2 out]
          }
          frame "MODBUS协议" {
            n159 = call "803M超标留样MB通讯.vi"("error in (no error)"=w346, "功能输入"=enum16{"打开串口", "写入", "读取", "关闭串口", "写入寄存器"}."关闭串口") -> ("error out"=w347:errorcluster)  [unwired: 8 in, 1 out]
          }
        }
      }
    }
  }
  n160 = call-by-ref "?"(reference=w11, error in=w9) -> (reference out=w8:refnum<vi>, error out=w7:errorcluster)  [unwired: 12 in]
  n161 = Close Reference(reference=w8, error in (no error)=w7) -> ()  [unwired: 1 out]
